vi "Append, Replace, Cancel or New.vi"(8 "NoNew":bool, 9 "NoCancel":bool, 10 "NoAppend":bool, 11 "PathIn":path=path "C:/TestText.dat") -> (0 "CancelOut":bool, 1 "ReplOut":bool, 2 "AppndOut":bool, 3 "PathOut":path, 4 "NewOut":bool)   [LabVIEW 2013]
doc: "Interacts with user and presents \"Append\", \"Replace\", \"New\" or \"Cancel\" options when doing a file write to a file which exists.\n\nAutoCon, 8/2002\n\nModififed 10/02 - added \"new file\" constant to frame 2:TRUE"
panel:
  out "Msg":string="exists - Append, Replace, Cancel or New ?"
  in  "New":bool
  in  "Append":bool
  in  "Replace":bool
  in  "Cancel":bool
  out "File:":string
  # "Warning - File exists"
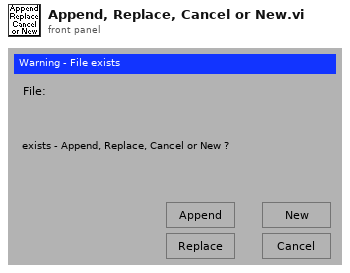
[diagram p1: front panel]
types:
  T1 = enum32{"existing file", "new file", "new or existing file", "existing dir", "new dir", "new or existing dir", "existing file (use LLBs)", "new file (use LLBs)", "new or existing file (use LLBs)", "new or existing file or directory (use LLBs)"}
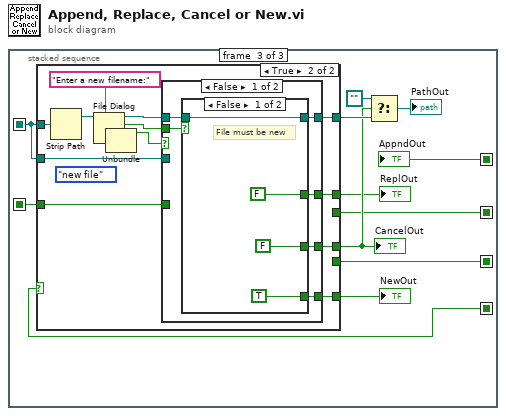
[diagram p0: block diagram]
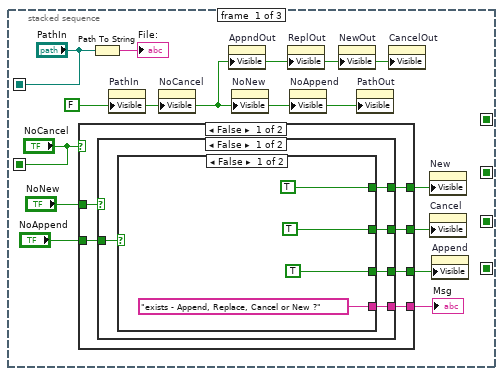
[diagram p2: hidden frame]
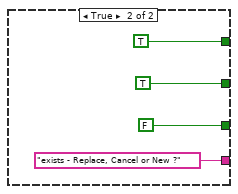
[diagram p3: hidden frame]
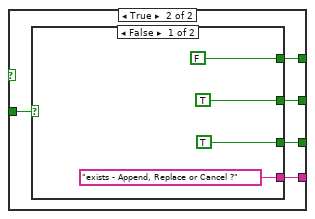
[diagram p4: hidden frame]
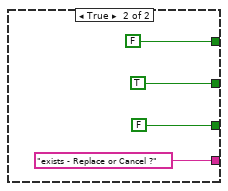
[diagram p5: hidden frame]
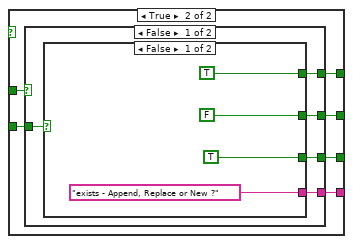
[diagram p6: hidden frame]
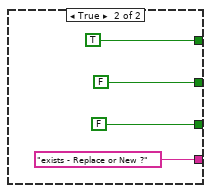
[diagram p7: hidden frame]
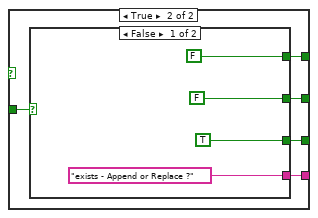
[diagram p8: hidden frame]
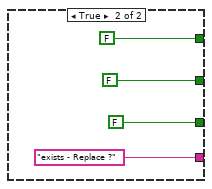
[diagram p9: hidden frame]
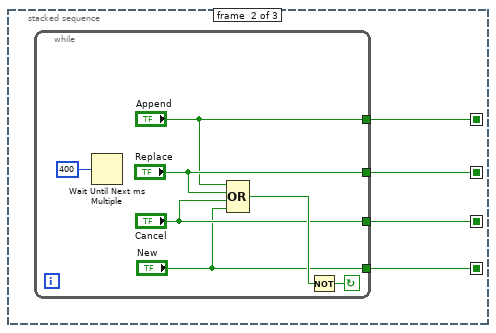
[diagram p10: hidden frame]
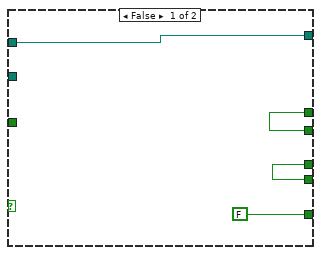
[diagram p11: hidden frame]
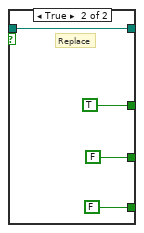
[diagram p12: hidden frame]
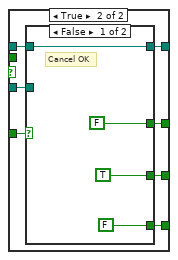
[diagram p13: hidden frame]
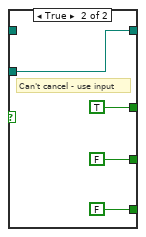
[diagram p14: hidden frame]
diagram:
  n1 = stacked-sequence {
    seq-local: ["PathIn" _ _] -> [_ _ w86]
    seq-local: [_ w78 _] -> [_ _ w94]
    seq-local: [_ w77 _] -> [_ _ w89]
    seq-local: [_ w76 _] -> [_ _ w92]
    seq-local: [_ w75 _] -> [_ _ w90]
    seq-local: ["NoCancel" _ _] -> [_ _ w87]
    frame #0 {
      w3 = FALSE ("Visible")
      n2 = case shown="False" "NoCancel" {
        tunnel: "NoNew" -> [w16 w48]
        tunnel: [w15 w46] -> w7
        tunnel: [w14 w47] -> w6
        tunnel: [w13 w45] -> w5
        tunnel: [w12 w44] -> w2
        tunnel: "NoAppend" -> [w11 w43]
        frame False {
          n3 = case shown="False" w16 {
            tunnel: [w21 w32] -> w15
            tunnel: [w20 w34] -> w14
            tunnel: [w19 w33] -> w13
            tunnel: [w18 w31] -> w12
            tunnel: w11 -> [w17 w30]
            frame False {
              n4 = case shown="False" w17 {
                tunnel: ["exists - Append, Replace, Cancel or New ?" ("Msg") "exists - Replace, Cancel or New ?" ("Msg")] -> w21
                tunnel: [TRUE TRUE] -> w20
                tunnel: [TRUE TRUE] -> w19
                tunnel: [TRUE FALSE] -> w18
                frame False {
                }
                frame True {
                }
              }
            }
            frame True {
              n5 = case shown="False" w30 {
                tunnel: [FALSE FALSE] -> w34
                tunnel: [TRUE TRUE] -> w33
                tunnel: ["exists - Append, Replace or Cancel ?" ("Msg") "exists - Replace or Cancel ?" ("Msg")] -> w32
                tunnel: [TRUE FALSE] -> w31
                frame False {
                }
                frame True {
                }
              }
            }
          }
        }
        frame True {
          n6 = case shown="False" w48 {
            tunnel: [w53 w66] -> w47
            tunnel: [w52 w64] -> w46
            tunnel: [w51 w65] -> w45
            tunnel: [w50 w62] -> w44
            tunnel: w43 -> [w49 w63]
            frame False {
              n7 = case shown="False" w49 {
                tunnel: [TRUE TRUE] -> w53
                tunnel: ["exists - Append, Replace or New ?" ("Msg") "exists - Replace or New ?" ("Msg")] -> w52
                tunnel: [FALSE FALSE] -> w51
                tunnel: [TRUE FALSE] -> w50
                frame False {
                }
                frame True {
                }
              }
            }
            frame True {
              n8 = case shown="False" w63 {
                tunnel: [FALSE FALSE] -> w66
                tunnel: [FALSE FALSE] -> w65
                tunnel: ["exists - Append or Replace ?" ("Msg") "exists - Replace ?" ("Msg")] -> w64
                tunnel: [TRUE FALSE] -> w62
                frame False {
                }
                frame True {
                }
              }
            }
          }
        }
      }
      "Msg" <- w7
      n9 = Path To String(path="PathIn") -> (string=→"File:":string)
      n10 = property on="PathIn" class="Path"("Visible"=w3) -> ()  [unwired: 2 in, 2 out]
      n11 = property on="NoCancel" class="Bool (strict)"("Visible"=w3) -> ()  [unwired: 2 in, 2 out]
      n12 = property on="AppndOut" class="Bool (strict)"("Visible"=w3) -> ()  [unwired: 2 in, 2 out]
      n13 = property on="NoNew" class="Bool (strict)"("Visible"=w3) -> ()  [unwired: 2 in, 2 out]
      n14 = property on="ReplOut" class="Bool (strict)"("Visible"=w3) -> ()  [unwired: 2 in, 2 out]
      n15 = property on="NoAppend" class="Bool (strict)"("Visible"=w3) -> ()  [unwired: 2 in, 2 out]
      n16 = property on="NewOut" class="Bool (strict)"("Visible"=w3) -> ()  [unwired: 2 in, 2 out]
      n17 = property on="PathOut" class="Path"("Visible"=w3) -> ()  [unwired: 2 in, 2 out]
      n18 = property on="CancelOut" class="Bool (strict)"("Visible"=w3) -> ()  [unwired: 2 in, 2 out]
      n19 = property on="New" class="Bool"("Visible"=w6) -> ()  [unwired: 2 in, 2 out]
      n20 = property on="Cancel" class="Bool"("Visible"=w5) -> ()  [unwired: 2 in, 2 out]
      n21 = property on="Append" class="Bool"("Visible"=w2) -> ()  [unwired: 2 in, 2 out]
    }
    frame #1 {
      n22 = while {
        tunnel: ["New"] -> w75
        tunnel: ["Cancel"] -> w76
        tunnel: ["Replace"] -> w77
        tunnel: ["Append"] -> w78
        stop <- w84 continue-if-true
        n23 = Wait Until Next ms Multiple(millisecond multiple=u32 400) -> ()  [unwired: 1 out]
        n24 = Compound Arithmetic op=OR("Append", "Replace", "Cancel", "New") -> (w83:bool)
        n25 = Not(x=w83) -> (.not. x?=w84:bool)
      }
    }
    frame #2 {
      n26 = case shown="True" w90 {
        tunnel: w86 -> [w101 w114]
        tunnel: [w101 w111] -> w96
        tunnel: [FALSE w113] -> w93
        tunnel: w92 -> [w99 _]
        tunnel: [w99 w112] -> w91
        tunnel: w89 -> [w98 _]
        tunnel: [w98 w106] -> w88
        tunnel: w87 -> [_ w104]
        tunnel: w86 -> [_ w103]
        frame False {
        }
        frame True {
          (unwired) T1."new file" ("select mode (2)")
          n27 = Strip Path(path=w114) -> (stripped path=w110:path)  [unwired: 1 out]
          n28 = File Dialog(7:"Enter a new filename:" ("prompt"), 11:w110) -> (0:w102:errorcluster, 1:w105:bool, 2:w107:bool, 3:w108:path)  [unwired: 5 in]
          n29 = Unbundle(w102) -> ()  [unwired: 3 out]
          n30 = case shown="False" w105 {
            tunnel: [w120 w130] -> w113
            tunnel: [w115 w131] -> w112
            tunnel: [w116 w133] -> w111
            tunnel: w108 -> [w117 w129]
            tunnel: w107 -> [w119 _]
            tunnel: [w118 w132] -> w106
            tunnel: w104 -> [_ w135]
            tunnel: w103 -> [_ w134]
            frame False {
              n31 = case shown="False" w119 {
                tunnel: [TRUE FALSE] -> w120
                tunnel: [FALSE TRUE] -> w118
                tunnel: w117 -> [w124 w127]
                tunnel: [w124 w127] -> w116
                tunnel: [FALSE FALSE] -> w115
                frame False {
                  # "File must be new"
                }
                frame True {
                  # "Replace"
                }
              }
            }
            frame True {
              n32 = case shown="False" w135 {
                tunnel: w134 -> [_ w143]
                tunnel: [w139 w143] -> w133
                tunnel: [FALSE TRUE] -> w132
                tunnel: [TRUE FALSE] -> w131
                tunnel: [FALSE FALSE] -> w130
                tunnel: w129 -> [w139 _]
                frame False {
                  # "Cancel OK"
                }
                frame True {
                  # "Can't cancel - use input"
                }
              }
            }
          }
        }
      }
      "CancelOut" <- w91
      "ReplOut" <- w88
      "NewOut" <- w93
      n33 = Select(t=path "", s=w91, f=w96) -> (s? t:f=→"PathOut":path)
      "AppndOut" <- w94
    }
  }
